vi "Read Commands.vi"(8 "error in (no error)":errorcluster, 11 "Relay in":refnum<class "Relay.lvclass">) -> (0 "error out":errorcluster, 2 "Commands":T1[](array[typedef]), 3 "Relay out":refnum<class "Relay.lvclass">)   [LabVIEW 2015, in "SLSC Switch.lvlib" / "Relay.lvclass"]
uses:
  Relay.lvclass
  Command.ctl
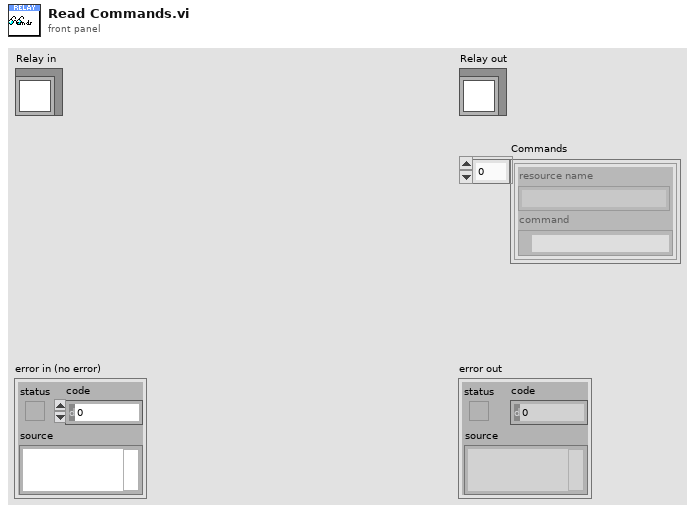
[diagram p1: front panel]
types:
  T1 = typedef "SLSC Switch.lvlib/Relay.lvclass/Command.ctl" = cluster{"resource name":string, "command":refnum<k21>}
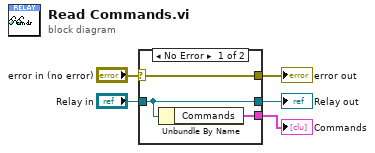
[diagram p0: block diagram]
diagram:
  n1 = case shown="No Error" "error in (no error)" {
    selector: "error in (no error)" -> [w8 w9]
    tunnel: [w8 w9] -> w4
    tunnel: [w7 w10] -> w2
    tunnel: "Relay in" -> [w7 w10]
    tunnel: [w6 _] -> w1
    frame No Error {
      n2 = Unbundle By Name(w7) -> ("Commands"=w6:T1[])
    }
    frame Error {
    }
  }
  "error out" <- w4
  "Relay out" <- w2
  "Commands" <- w1
